vi "0xE2_Cmd_write_one_parameter_of_type_int_(SubVI).vi"(9 "Значение параметра":i32, 10 "Номер параметра":i32, 11 "String in":string) -> (3 "String out":string)   [LabVIEW 2017, in "LV_Unicorn.lvlib"]
uses:
  LV_Unicorn.lvlib
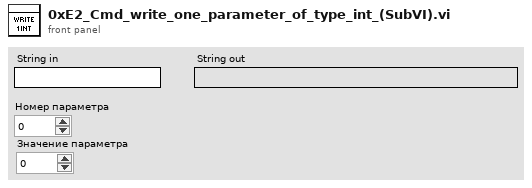
[diagram p1: front panel]
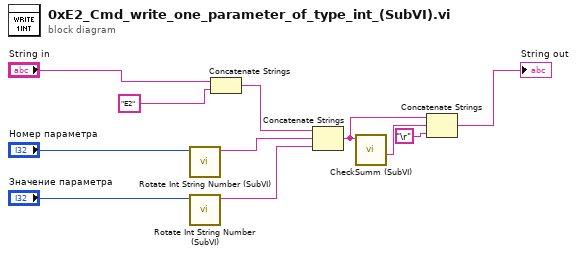
[diagram p0: block diagram]
diagram:
  n1 = call "Rotate Int String Number (SubVI).vi"("Int Number In"="Номер параметра") -> ("Orig String"=w3:string)  [unwired: 8 in, 2 out]
  n2 = call "Rotate Int String Number (SubVI).vi"("Int Number In"="Значение параметра") -> ("Orig String"=w4:string)  [unwired: 8 in, 2 out]
  n3 = Concatenate Strings("String in", "E2" ("string")) -> (w9:string)
  n4 = Concatenate Strings(w9, w3, w4) -> (w6:string)
  n5 = call "CheckSumm (SubVI).vi"("Input String"=w6) -> ("CheckSumm"=w5:string)  [unwired: 7 in, 3 out]
  n6 = Concatenate Strings(w6, w5, "\r") -> (→"String out":string)
